vi "Get Click Location.vi"(8 "error in (no error)":errorcluster, 9 "Coords":T1, 10 "Tree Refnum":refnum<vi>, 11 "Tree Click Interpreter in":refnum<class "Tree Click Interpreter.lvclass">) -> (0 "error out":errorcluster, 1 "Valid?":bool, 2 "Insertion Index":i32, 3 "Parent ID":string, 5 "Tag":string)   [LabVIEW 2017, in "Tree Click Interpreter.lvclass"]
uses:
  <vilib>/gpm_packages/@cs/Test-executive-builder/Source/Test Executive Builder View/Tree Click Interpreter/Tree Click Interpreter.lvclass
  <vilib>/Utility/miscctls.llb/LVPoint32TypeDef.ctl
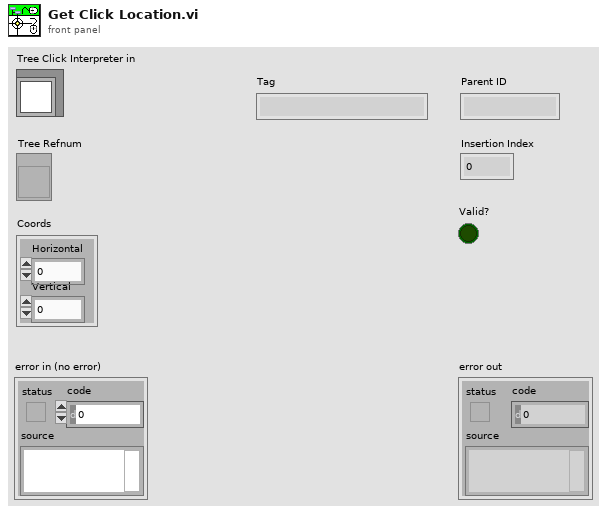
[diagram p1: front panel]
types:
  T1 = typedef "LVPoint32TypeDef.ctl" = cluster{"Horizontal":i32, "Vertical":i32}
  T2 = typedef "Relative Click Location.ctl" = enum16{"Unknown Location", "Below Element", "On Element", "Above Element"}
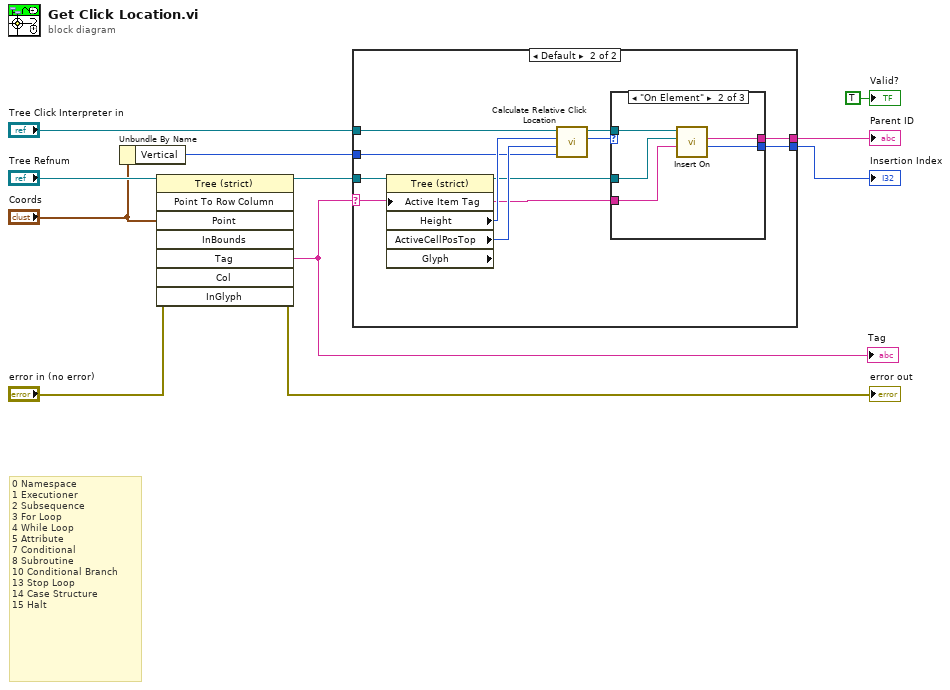
[diagram p0: block diagram]
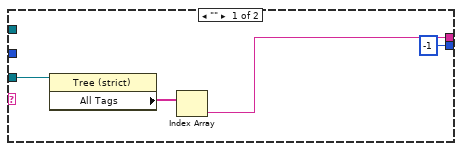
[diagram p2: hidden frame]
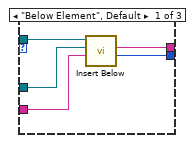
[diagram p3: hidden frame]
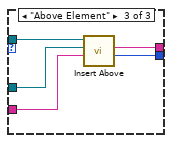
[diagram p4: hidden frame]
diagram:
  # "0 Namespace\n1 Executioner\n2 Subsequence\n3 For Loop\n4 While Loop\n5 Attribute\n7 Conditional\n8 Subroutine\n10 Conditional Branch\n13 Stop Loop\n14 Case Structure\n15 Halt"
  n1 = Unbundle By Name("Coords") -> ("Vertical"=w3:i32)
  n2 = invoke class="Tree (strict)" method="Point To Row Column"(reference="Tree Refnum", error in="error in (no error)", "Point"="Coords") -> (reference out=w6:refnum<vi>, error out=→"error out":errorcluster, "Tag"=w2:string)  [unwired: 5 in, 5 out]
  "Tag" <- w2
  n3 = case shown="Default" w2 {
    selector: w2 -> [_ w17]
    tunnel: [w13 w26] -> w10
    tunnel: [-1 ("Insertion Index") w25] -> w9
    tunnel: w6 -> [w15 w24]
    tunnel: "Tree Click Interpreter in" -> [_ w23]
    tunnel: w3 -> [_ w19]
    frame "" {
      n4 = property class="Tree (strict)"(reference=w15) -> ("All Tags"=w14:string[])  [unwired: 1 in, 2 out]
      n5 = Index Array(array=w14) -> (element=w13:string)  [unwired: 1 in]
    }
    frame Default {
      n6 = property class="Tree (strict)" props=["Active Item Tag", "Height", "ActiveCellPosTop", "Glyph"](reference=w24, "Active Item Tag"=w17) -> (reference out=w18:refnum<vi>, "Height"=w21:i32, "ActiveCellPosTop"=w20:i32)  [unwired: 1 in, 2 out]
      n7 = call-dynamic "Calculate Relative Click Location.vi"("Click Vertical Position"=w19, "Cell Top Position"=w20, "Cell Height"=w21, "Tree Click Interpreter in"=w23) -> ("Relative Click Location"=w16:T2, "Tree Click Interpreter out"=w22:refnum<class "Tree Click Interpreter.lvclass">)  [unwired: 6 in]
      n8 = case shown="\"On Element\"" w16 {
        tunnel: [w31 w33 w40] -> w26
        tunnel: [w30 w32 w39] -> w25
        tunnel: w22 -> [w29 w36 w41]
        tunnel: w18 -> [w28 w35 w38]
        tunnel: w17 -> [w27 w34 w37]
        frame "Below Element", Default {
          n9 = call-dynamic "Insert Below.vi"("Item Tag"=w27, "Tree Refnum"=w28, "Tree Click Interpreter in"=w29) -> ("Insertion Index"=w30:i32, "Parent ID"=w31:string)  [unwired: 5 in, 2 out]
        }
        frame "On Element" {
          n10 = call-dynamic "Insert On.vi"("Item Tag"=w34, "Tree Refnum"=w35, "Tree Click Interpreter in"=w36) -> ("Insertion Index"=w32:i32, "Parent ID"=w33:string)  [unwired: 5 in, 2 out]
        }
        frame "Above Element" {
          n11 = call-dynamic "Insert Above.vi"("Item Tag"=w37, "Tree Refnum"=w38, "Tree Click Interpreter in"=w41) -> ("Insertion Index"=w39:i32, "Parent ID"=w40:string)  [unwired: 5 in, 2 out]
        }
      }
    }
  }
  "Parent ID" <- w10
  "Insertion Index" <- w9
  "Valid?" <- TRUE ("Valid?")
